vi "Post-Register.vi"(8 "error in (no error)":errorcluster, 11 "Report Generator in":refnum<class "Report Generator.lvclass">) -> (0 "error out":errorcluster, 3 "Report Generator out":refnum<class "Report Generator.lvclass">)   [LabVIEW 2023, in "Report Generator.lvlib" / "Report Generator.lvclass"]
doc: "<b>Post Register</b>\nThis routine is implemented in <b>Post Launch Initialize</b> after the actor has registered for events.\n\nIt's intended to provide a means of performing actions immediately before the actor state engine is entered.\n\n<b>Report Generator</b> Create a 10Hz flush report queue message to process all buffered data in the report queue."
uses:
  Library/Report Generator.lvclass
  Library/Report Generator.lvclass/Report Generator.ctl
  Report Generator Messages/Periodically Flush Queue Msg/Periodically Flush Queue Msg.lvclass
  builds/Framework/Actor Framework.lvlibp
  C:/Users/Public/Documents/Development/builds/Framework/Actor Framework.lvlibp/1abvi3w/vi.lib/ActorFramework/Message/Message.lvclass
  C:/Users/Public/Documents/Development/Application/Prime Panels/Report Generator/Report Generator Messages/Periodically Flush Queue Msg/Periodically Flush Queue Msg.lvclass
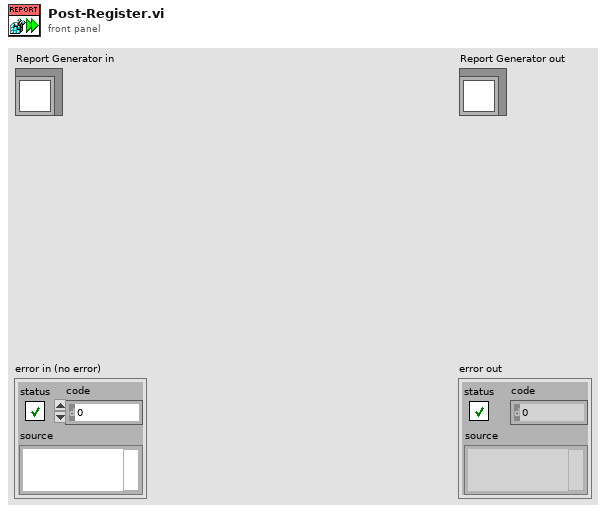
[diagram p1: front panel]
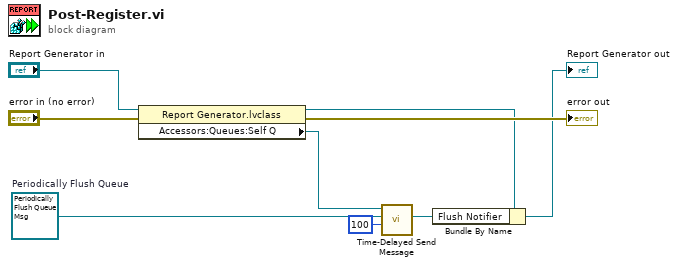
[diagram p0: block diagram]
diagram:
  w4 = refnum<class "Periodically Flush Queue Msg.lvclass"> refnum  # Periodically Flush Queue
  n1 = property class="Report Generator.lvclass"(reference="Report Generator in", error in="error in (no error)") -> (reference out=w6:refnum<class "Report Generator.lvclass">, error out=→"error out":errorcluster, "Accessors:Queues:Self Q"=w5:refnum<class "Message Enqueuer.lvclass">)
  n2 = call "Time-Delayed Send Message.vi"("Milliseconds To Wait"=100, "Message"=w4, "Message Enqueuer"=w5) -> ("Delivery Notifier"=w1:refnum<notifier>)  [unwired: 7 in, 1 out]
  n3 = Bundle By Name(cluster=w6, "Flush Notifier"=w1) -> (→"Report Generator out":refnum<class "Report Generator.lvclass">)
